vi "Saveconfig_MB.vi"(0 "configuration file path":path, 3 "Configuracion":cluster{bool[], u32[], string[], dbl[]}) -> (5 "error out":errorcluster)   [LabVIEW 2015]
uses:
  <vilib>/Utility/config.llb/Write Key (Double).vi
  <vilib>/Utility/config.llb/Write Key (String).vi
  <vilib>/Utility/config.llb/Write Key (U32).vi
  <vilib>/Utility/config.llb/Write Key (Boolean).vi
  <vilib>/Utility/config.llb/NI_LVConfig.lvlib
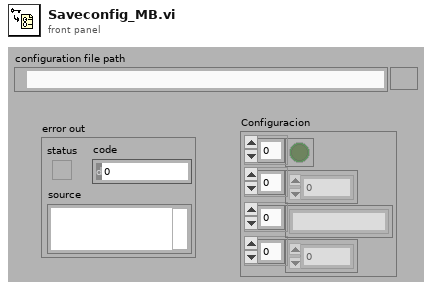
[diagram p1: front panel]
types:
  T1 = typedef "NI_LVConfig.lvlib/Config Data RefNum.ctl" = refnum<k1>
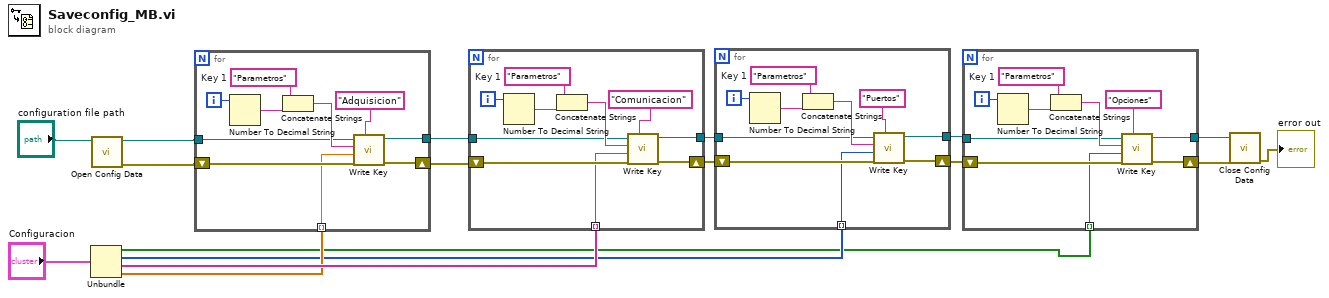
[diagram p0: block diagram]
diagram:
  n1 = Unbundle("Configuracion") -> (w1:bool[], w2:u32[], w7:string[], w3:dbl[])
  n2 = call <vilib>:"Open Config Data.vi"("configuration file path"="configuration file path") -> ("error out"=w8:errorcluster, "refnum"=w9:T1)  [unwired: 2 in, 7 out]
  n3 = for {
    tunnel: w9 -> [w22]
    tunnel: w3 -> [w20] mode=indexing
    shift-right: [w19] -> w4
    shift-left: w8 -> [w21]
    tunnel: [w18] -> w5
    i -> [w26]
    w24 = "Parametros"  # Key 1
    n4 = Number To Decimal String(number=w26) -> (decimal integer string=w25:string)  [unwired: 1 in]
    n5 = Concatenate Strings(w24, w25) -> (w23:string)
    n6 = call-poly <vilib>:"Write Key.vi"("section"="Adquisicion", "error in (no error)"=w21, "value"=w20, "key"=w23, "refnum"=w22) -> ("error out"=w19:errorcluster, "refnum out"=w18:T1)  [unwired: 3 in, 2 out]
  }
  n7 = for {
    tunnel: w5 -> [w32]
    tunnel: w7 -> [w28] mode=indexing
    shift-right: [w30] -> w12
    shift-left: w4 -> [w31]
    tunnel: [w29] -> w11
    i -> [w36]
    w34 = "Parametros"  # Key 1
    n8 = Number To Decimal String(number=w36) -> (decimal integer string=w35:string)  [unwired: 1 in]
    n9 = Concatenate Strings(w34, w35) -> (w33:string)
    n10 = call-poly <vilib>:"Write Key.vi"("section"="Comunicacion", "error in (no error)"=w31, "value"=w28, "key"=w33, "refnum"=w32) -> ("error out"=w30:errorcluster, "refnum out"=w29:T1)  [unwired: 1 in, 4 out]
  }
  n11 = for {
    tunnel: w11 -> [w42]
    tunnel: w2 -> [w38] mode=indexing
    shift-right: [w40] -> w14
    shift-left: w12 -> [w41]
    tunnel: [w39] -> w13
    i -> [w46]
    w44 = "Parametros"  # Key 1
    n12 = Number To Decimal String(number=w46) -> (decimal integer string=w45:string)  [unwired: 1 in]
    n13 = Concatenate Strings(w44, w45) -> (w43:string)
    n14 = call-poly <vilib>:"Write Key.vi"("section"="Puertos", "error in (no error)"=w41, "value"=w38, "key"=w43, "refnum"=w42) -> ("error out"=w40:errorcluster, "refnum out"=w39:T1)  [unwired: 5 out]
  }
  n15 = for {
    tunnel: w13 -> [w52]
    tunnel: w1 -> [w48] mode=indexing
    shift-right: [w50] -> w16
    shift-left: w14 -> [w51]
    tunnel: [w49] -> w15
    i -> [w56]
    w54 = "Parametros"  # Key 1
    n16 = Number To Decimal String(number=w56) -> (decimal integer string=w55:string)  [unwired: 1 in]
    n17 = Concatenate Strings(w54, w55) -> (w53:string)
    n18 = call-poly <vilib>:"Write Key.vi"("section"="Opciones", "error in (no error)"=w51, "value"=w48, "key"=w53, "refnum"=w52) -> ("error out"=w50:errorcluster, "refnum out"=w49:T1)  [unwired: 5 out]
  }
  n19 = call <vilib>:"Close Config Data.vi"("error in (no error)"=w16, "refnum"=w15) -> ("error out"=→"error out":errorcluster)  [unwired: 8 in, 1 out]
